vi "Test Controller To Terminate on Timeout when Verification Failed.vi"(8 "error in (no error)":errorcluster, 11 "Test Case In":refnum<class "Controller Test.lvclass">) -> (0 "error out":errorcluster, 3 "Test Case Out":refnum<class "Controller Test.lvclass">)   [LabVIEW 2020, in "Controller Test.lvclass"]
uses:
  Controller Test.lvclass
  Controller Test.lvclass/Controller Test.ctl
  01074fa8-ee8a-411d-bc8b-fc92c4f90959.vi
  ATM Controller/ATM Controller.lvclass
  ATM Controller/State.ctl
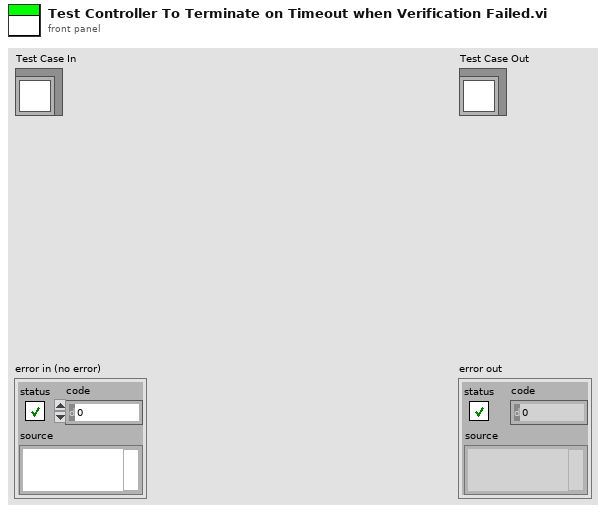
[diagram p1: front panel]
types:
  T1 = typedef "ATM Controller.lvclass/State.ctl" = enum16{"Start", "Card Inserted", "Verification Failed", "Verification Succeeded", "Terminate"}
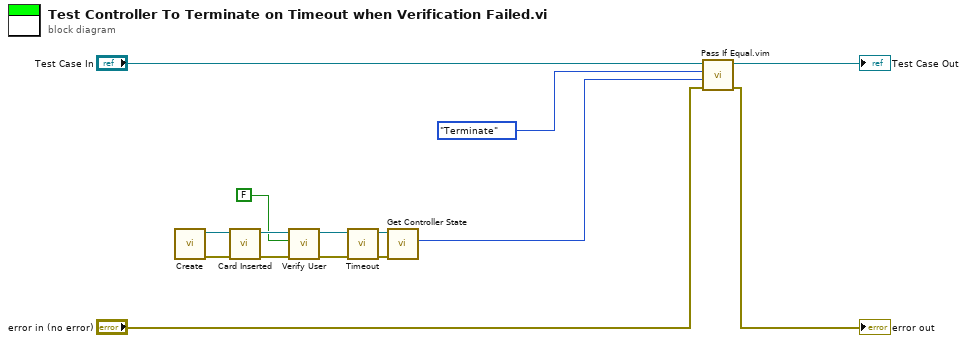
[diagram p0: block diagram]
diagram:
  n1 = call "Create.vi"() -> ("error out"=w11:errorcluster, "ATM Controller out"=w5:refnum<class "ATM Controller.lvclass">)  [unwired: 10 in]
  n2 = call "Card Inserted.vi"("error in (no error)"=w11, "ATM Controller in"=w5) -> ("error out"=w6:errorcluster, "ATM Controller out"=w3:refnum<class "ATM Controller.lvclass">)  [unwired: 8 in]
  n3 = call "Verify User.vi"("error in (no error)"=w6, "Verified?"=FALSE, "ATM Controller in"=w3) -> ("error out"=w4:errorcluster, "ATM Controller out"=w2:refnum<class "ATM Controller.lvclass">)  [unwired: 7 in]
  n4 = call "Timeout.vi"("error in (no error)"=w4, "ATM Controller in"=w2) -> ("error out"=w8:errorcluster, "ATM Controller out"=w7:refnum<class "ATM Controller.lvclass">)  [unwired: 8 in]
  n5 = call "Get Controller State.vi"("error in (no error)"=w8, "ATM Controller in"=w7) -> ("ATM State"=w10:T1)  [unwired: 7 in, 2 out]
  n6 = call "Pass If Equal.vim"("error in (no error)"="error in (no error)", "Actual"=w10, "Expected"=State."Terminate" ("ATM State"), "LUnit Test Case In"="Test Case In") -> ("error out"=→"error out":errorcluster, "LUnit Test Case Out"=→"Test Case Out":refnum<class "Controller Test.lvclass">)  [unwired: 6 in]
